vi "MACBIN VI Tree__ogtk.vi"() -> ()   [LabVIEW 2018]
uses:
  <userlib>/_OpenG.lib/lvzip/macbin.llb/MACBIN Macbinary Header__ogtk.ctl
  <userlib>/_OpenG.lib/lvzip/macbin.llb/MACBIN Resource Header__ogtk.ctl
panel:
  in  "finder info":T1 {"mod date" format="%<%H:%M:%S\n%m/%d/%Y>T"; "creation date" format="%<%H:%M:%S\n%m/%d/%Y>T"}
  in  "macbinary header":T2 {"last mod" format="%<%I:%M:%S %p\n%d/%m/%y>T"; "creation date" format="%<%H:%M:%S\n%d/%m/%y>T"}
  # "Please visit http://www.OpenG.org to learn about the\nOpen Source LabVIEW software movement.\n\nNOTICE -- YOU MUST LEAVE THIS NOTICE IN PLACE.  PER THE TERMS OF THE LICENSE BELOW, YOU MAY SUBLICENSE THIS SOFTWARE \nIN ANY WAY THAT DOES NOT CONFLICT WITH THIS LICENSE.\n\n### BSD License (http://www.opensource.org/licenses/bsd-license.php) Begin ###\n \nCopyright (C) 2002 Christophe Salzmann christophe.salzmann@epfl.ch\nCopyright (C) 2002-2006 Rolf Kalbermatter rolf.kalbermatter@citengineering.com\n\nAll rights reserved.\n\nRedistribution and use in source and binary forms, with or without modification, are permitted provided that the following conditions are met:\n\n    * Redistributions of source code must retain the above copyright notice, this list of conditions and the following disclaimer.\n    * Redistributions in binary form must reproduce the above copyright notice, this list of conditions and the following disclaimer in the \n       documentation and/or other materials provided with the distribution.\n    * Neither the name of SciWare, James Kring, Inc., nor the names of its contributors may be used to endorse or promote products derived \n       from this software without specific prior written permission.\n\nTHIS SOFTWARE IS PROVIDED BY THE COPYRIGHT HOLDERS AND CONTRIBUTORS \"AS IS\" AND ANY EXPRESS OR IMPLIED WARRANTIES, \nINCLUDING, BUT NOT LIMITED TO, THE IMPLIED WARRANTIES OF MERCHANTABILITY AND FITNESS FOR A PARTICULAR PURPOSE ARE \nDISCLAIMED. IN NO EVENT SHALL THE COPYRIGHT OWNER OR CONTRIBUTORS BE LIABLE FOR ANY DIRECT, INDIRECT, INCIDENTAL,\n SPECIAL, EXEMPLARY, OR CONSEQUENTIAL DAMAGES (INCLUDING, BUT NOT LIMITED TO, PROCUREMENT OF SUBSTITUTE GOODS OR \nSERVICES; LOSS OF USE, DATA, OR PROFITS; OR BUSINESS INTERRUPTION) HOWEVER CAUSED AND ON ANY THEORY OF LIABILITY, \nWHETHER IN CONTRACT, STRICT LIABILITY, OR TORT (INCLUDING NEGLIGENCE OR OTHERWISE) ARISING IN ANY WAY OUT OF THE USE \nOF THIS SOFTWARE, EVEN IF ADVISED OF THE POSSIBILITY OF SUCH DAMAGE.\n\n### BSD License End ###"
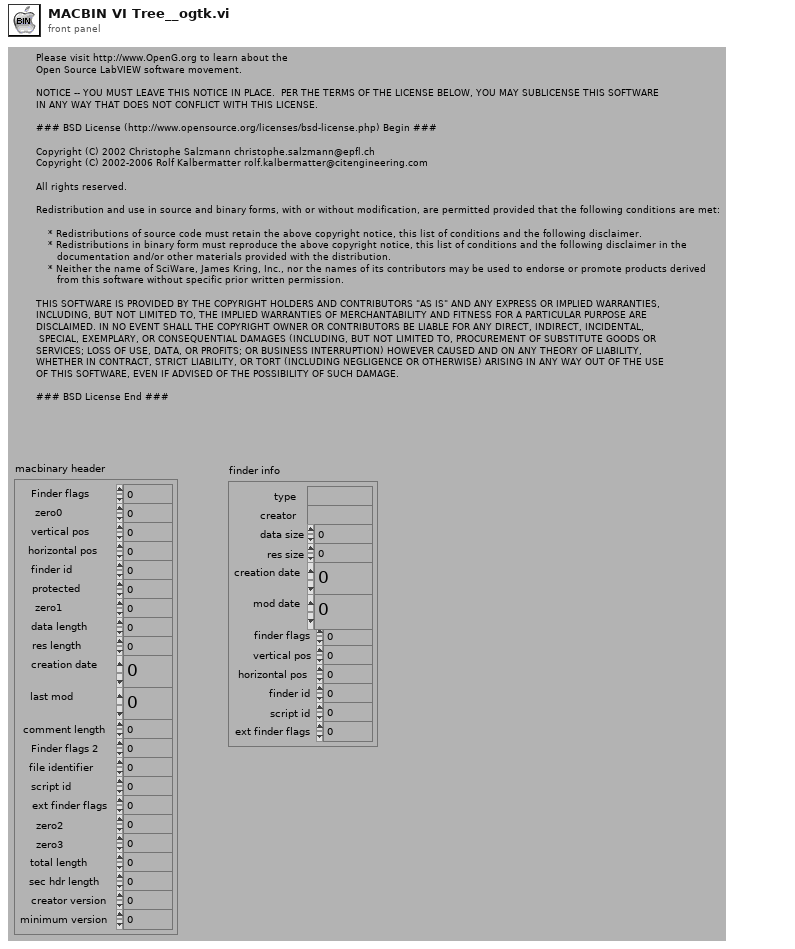
[diagram p1: front panel]
types:
  T1 = typedef "MACBIN Resource Header__ogtk.ctl" = cluster{"type":string, "creator":string, "data size":u32, "res size":u32, "creation date":u32, "mod date":u32, "finder flags":u16, "vertical pos":i16, "horizontal pos":i16, "finder id":u16, "script id":u8, "ext finder flags":u8}
  T2 = typedef "MACBIN Macbinary Header__ogtk.ctl" = cluster{"Finder flags":u8, "zero0":u8, "vertical pos":u16, "horizontal pos":u16, "finder id":u16, "protected":u8, "zero1":u8, "data length":i32, "res length":i32, "creation date":u32, "last mod":u32, "comment length":i16, "Finder flags 2":u8, "file identifier":u32, "script id":u8, "ext finder flags":u8, "zero2":i32, "zero3":i32, "total length":u32, "sec hdr length":u16, "creator version":u8, "minimum version":u8}
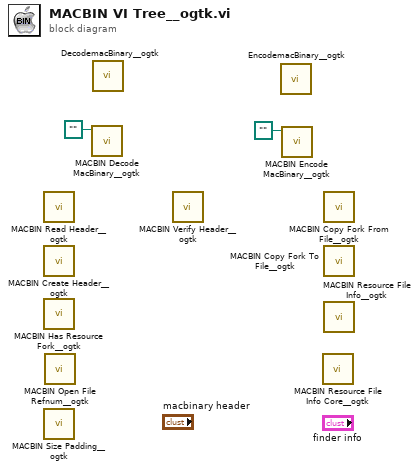
[diagram p0: block diagram]
diagram:
  n1 = call <userlib>:"MACBIN Read Header__ogtk.vi"() -> ()  [unwired: 4 in, 6 out]
  n2 = call <userlib>:"MACBIN Create Header__ogtk.vi"() -> ()  [unwired: 4 in, 7 out]
  n3 = call <userlib>:"MACBIN Has Resource Fork__ogtk.vi"() -> ()  [unwired: 5 in, 3 out]
  n4 = call <userlib>:"MACBIN Size Padding__ogtk.vi"() -> ()  [unwired: 5 in, 1 out]
  n5 = call <userlib>:"MACBIN Open File Refnum__ogtk.vi"() -> ()  [unwired: 7 in, 2 out]
  n6 = call <userlib>:"MACBIN Decode MacBinary__ogtk.vi"("macbinary file"=path "") -> ()  [unwired: 3 in, 4 out]
  n7 = call <userlib>:"DecodemacBinary__ogtk.vi"() -> ()  [unwired: 11 in, 1 out]
  n8 = call <userlib>:"MACBIN Verify Header__ogtk.vi"() -> ()  [unwired: 5 in, 7 out]
  n9 = call <userlib>:"EncodemacBinary__ogtk.vi"() -> ()  [unwired: 11 in, 1 out]
  n10 = call <userlib>:"MACBIN Encode MacBinary__ogtk.vi"("data file"=path "" ("macbinary file")) -> ()  [unwired: 3 in, 4 out]
  n11 = call <userlib>:"MACBIN Resource File Info Core__ogtk.vi"() -> ()  [unwired: 5 in, 5 out]
  n12 = call <userlib>:"MACBIN Copy Fork From File__ogtk.vi"() -> ()  [unwired: 6 in, 3 out]
  n13 = call <userlib>:"MACBIN Copy Fork To File__ogtk.vi"() -> ()  [unwired: 6 in, 3 out]
  n14 = call <userlib>:"MACBIN Resource File Info__ogtk.vi"() -> ()  [unwired: 7 in, 5 out]
